vi "TestRFGVBedVacant.vi"() -> (2 "Pass":bool)   [LabVIEW 2015]
uses:
  NurseStation/TypeDef/SelectedRoom.ctl
  LVClasses/Flags/ColorFlags.ctl
  TypeDef/RoomsActionEnum.ctl
  LVClasses/Room/Room.lvclass
  LVClasses/Flags/Flags.lvclass
panel:
  out "Selected Room":T1={"Room Number"=0, "RoomNumFlags"={"Flag State"=[1, 3, 5, 7]}, "BedVacant"=FALSE, "InRoomPersonnel"=[], "RoomRequests"=[]}
  out "error out":errorcluster
  out "JSON string":string
  out "Read 2":string
  out "Read1":string
  in  "BedVacant":bool
  out "Write":string
  in  "FGV Room":i32=102
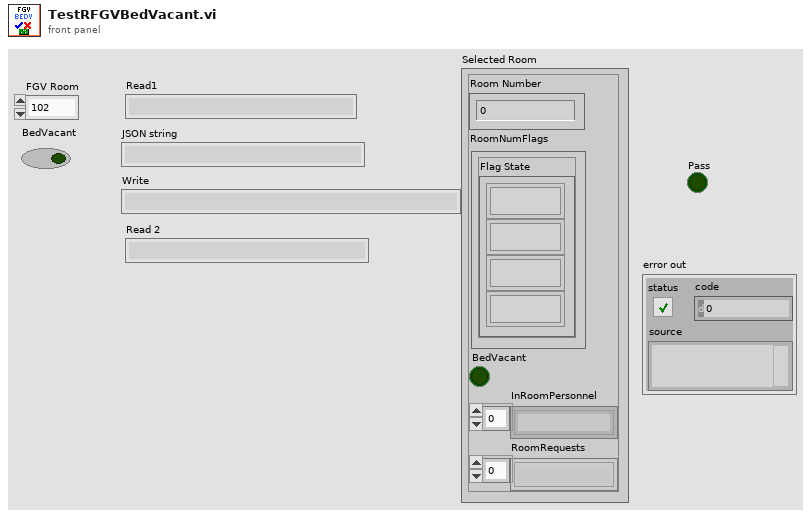
[diagram p1: front panel]
types:
  T1 = typedef "SelectedRoom.ctl" = cluster{"Room Number":u8, "RoomNumFlags":T2, "BedVacant":bool, "InRoomPersonnel":string[], "RoomRequests":string[]}
  T2 = typedef "Flags.lvclass/ColorFlags.ctl" = cluster{"Flag State":u8[]}
  T3 = typedef "RoomsActionEnum.ctl" = enum16{"Init", "Add Room", "Remove Room", "Read Room", "Read Flag", "Read Flag State", "Write Flag State", "Read Flag Color", "Write Flag Color", "Read Bed Vacant", "Write Bed Vacant", "Read Personnel", "Add Personnel", "Remove Personnel", "Read Requests", "Add Request", "Remove Request", "Read Beacon ID", "Write Beacon ID", "Write Bed URL", "Read Bed URL", "Read Rooms Numbers", "Write Flag"}
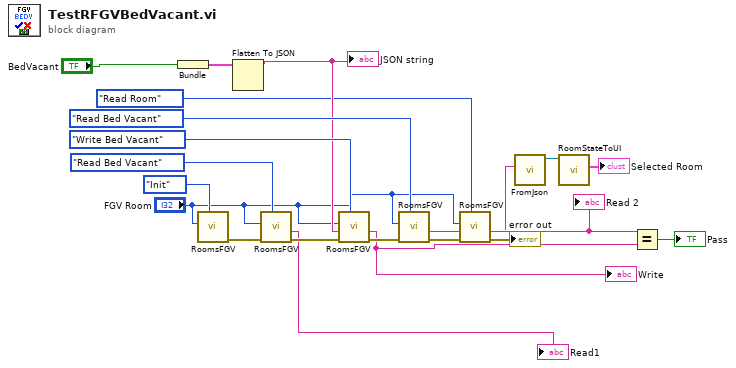
[diagram p0: block diagram]
diagram:
  n1 = Bundle("BedVacant"="BedVacant") -> (w11:cluster{"BedVacant":bool})  [unwired: 1 in]
  n2 = call "RoomsFGV.vi"("Actions"=RoomsActionEnum."Init", "Room"="FGV Room") -> ("error out"=w20:errorcluster)  [unwired: 8 in, 1 out]
  n3 = Flatten To JSON(anything=w11) -> (JSON string=w10:string)  [unwired: 2 in, 1 out]
  "JSON string" <- w10
  n4 = call "RoomsFGV.vi"("Actions"=RoomsActionEnum."Read Bed Vacant", "error in (no error)"=w20, "Room"="FGV Room") -> ("error out"=w19:errorcluster, "Data Out"=→"Read1":string)  [unwired: 7 in]
  n5 = call "RoomsFGV.vi"("Actions"=RoomsActionEnum."Write Bed Vacant", "error in (no error)"=w19, "Data In"=w10, "Room"="FGV Room") -> ("error out"=w18:errorcluster, "Data Out"=w8:string)  [unwired: 6 in]
  "Write" <- w8
  n6 = call "RoomsFGV.vi"("Actions"=RoomsActionEnum."Read Bed Vacant", "error in (no error)"=w18, "Room"="FGV Room") -> ("error out"=w7:errorcluster, "Data Out"=w9:string)  [unwired: 7 in]
  "Read 2" <- w9
  n7 = call "RoomsFGV.vi"("Actions"=RoomsActionEnum."Read Room", "error in (no error)"=w7, "Room"="FGV Room") -> ("error out"=→"error out":errorcluster, "Data Out"=w1:string)  [unwired: 7 in]
  n8 = call "FromJson.vi"("String"=w1) -> ("Room out"=w3:refnum<class "Room.lvclass">)  [unwired: 9 in, 1 out]
  n9 = call "RoomStateToUI.vi"("Room In"=w3) -> ("Selected Room"=→"Selected Room":T1)  [unwired: 8 in, 2 out]
  n10 = Equal?(x=w9, y=w8) -> (x = y?=→"Pass":bool)
